vi "SelectAppInstance.vi"(8 "error in":errorcluster, 11 "Application Reference (in)":refnum<vi>) -> (0 "error out":errorcluster, 1 "User Selected an App Instance?":bool, 2 "App Instance Ring (out)":u16(ring) items=["Default Application Instance"], 3 "Application Reference (out)":refnum<vi>)   [LabVIEW 2013, in "DiscoverCommonTypeDefCallers.lvlib"]
doc: "Outputs a valid application reference if one is provided as input; otherwise, prompts the user to select which existing application instance they wish work with. This provides a mechanism for running the calling VI either stand-alone, or by calling it from its own parent VI which has already determined the proper application reference."
uses:
  DiscoverCommonTypeDefCallers.lvlib
  LVTM.lvlib
panel:
  in  "OK Button":bool
  in  "Select App Instance":u16(ring) items=["Default Application Instance", "Task Manager.lvproj:My Computer", "LVTM_Tim.lvproj:My Computer"]
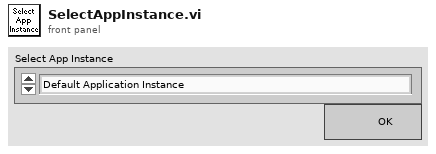
[diagram p1: front panel]
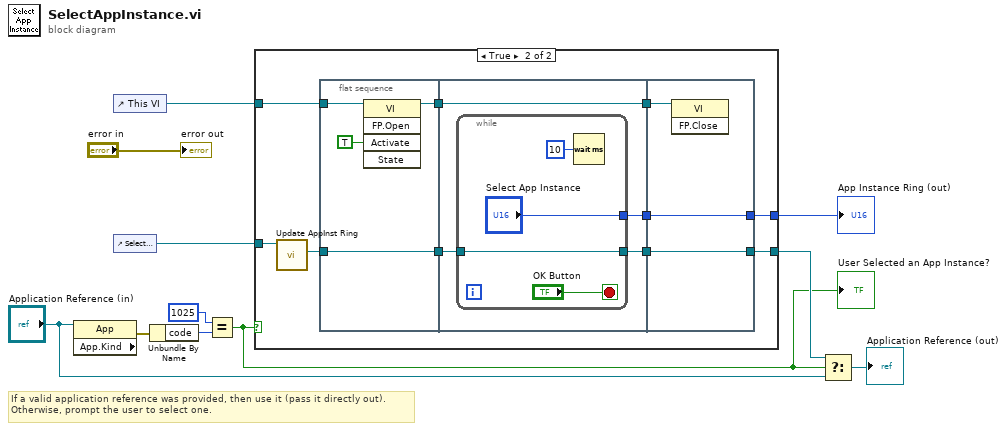
[diagram p0: block diagram]
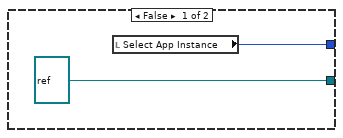
[diagram p2: hidden frame]
diagram:
  # "If a valid application reference was provided, then use it (pass it directly out).\nOtherwise, prompt the user to select one."
  n1 = property class="App" props=["App.Kind"](reference="Application Reference (in)") -> (error out=w6:errorcluster)  [unwired: 1 in, 2 out]
  n2 = control-ref of="This VI"() -> (w7:refnum<vi>)
  n3 = control-ref of="Select App Instance"() -> (w9:refnum<vi>)
  n4 = Unbundle By Name(w6) -> ("code"=w4:i32)
  n5 = Equal?(x=1025 ("Code to filter"), y=w4) -> (x = y?=w3:bool)
  "User Selected an App Instance?" <- w3
  n6 = case shown="True" w3 {
    tunnel: [refnum<vi> refnum ("AppInst out") w22] -> w10
    tunnel: w9 -> [_ w23]
    tunnel: [w12 w20] -> w8
    tunnel: w7 -> [_ w16]
    frame False {
      n7 = local read "Select App Instance"() -> (w12:u16)
    }
    frame True {
      n8 = call "Update AppInst Ring.vi"("Ring in"=w23) -> ("AppInst out"=w21:refnum<vi>)  [unwired: 8 in, 2 out]
      n9 = flat-sequence {
        tunnel: w21 -> [w27]
        tunnel: [w27] -> w19
        tunnel: w16 -> [w24]
        tunnel: [w25] -> w14
        tunnel: w19 -> [w30]
        tunnel: [w31] -> w18
        tunnel: [w29] -> w17
        tunnel: [w28] -> w15
        tunnel: w14 -> [w28]
        tunnel: [w37] -> w20
        tunnel: [w38] -> w22
        tunnel: w18 -> [w38]
        tunnel: w17 -> [w37]
        tunnel: w15 -> [w36]
        frame #0 {
          n10 = invoke class="VI" method="FP.Open"(reference=w24, "Activate"=TRUE ("Activate?")) -> (reference out=w25:refnum<vi>)  [unwired: 3 in, 4 out]
        }
        frame #1 {
          n11 = while {
            tunnel: [w34] -> w31
            tunnel: w30 -> [w34]
            tunnel: ["Select App Instance"] -> w29
            stop <- "OK Button" stop-if-true
            n12 = Wait (ms)(milliseconds to wait=u32 10) -> ()  [unwired: 1 out]
          }
        }
        frame #2 {
          n13 = invoke class="VI" method="FP.Close"(reference=w36) -> ()  [unwired: 2 in, 3 out]
        }
      }
    }
  }
  "App Instance Ring (out)" <- w8
  n14 = Select(t=w10, s=w3, f="Application Reference (in)") -> (s? t:f=→"Application Reference (out)":refnum<vi>)
  "error out" <- "error in"
